vi "Send to HTTP Manager.vi"(8 "error in (no error)":errorcluster, 9 "Data":variant, 10 "ID":string, 11 "VolatusAPI in":refnum<class "VolatusAPI.lvclass">) -> (0 "error out":errorcluster, 3 "VolatusAPI out":refnum<class "VolatusAPI.lvclass">)   [LabVIEW 2020, in "Volatus.lvlib" / "VolatusAPI.lvclass"]
uses:
  VolatusAPI.lvclass
  VolatusAPI.lvclass/VolatusAPI.ctl
  MessageQ/MessageQ.lvclass
  HTTP Manager Identity/HTTP Manager Identity.lvclass
  C:/dev/lv20CE/relink/lv-volatus/Volatus/HTTP Manager Identity/HTTP Manager Identity.lvclass
  C:/dev/lv20CE/relink/lv-volatus/Volatus/Identity/Identity.lvclass
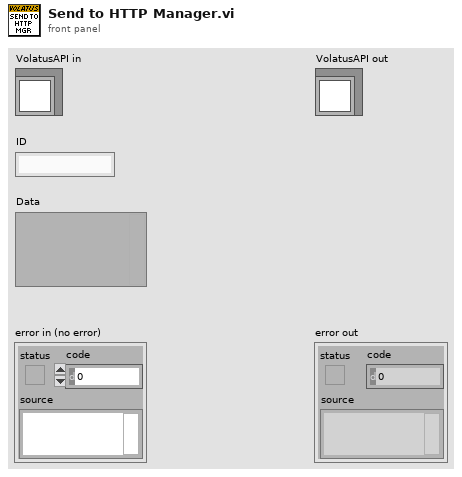
[diagram p1: front panel]
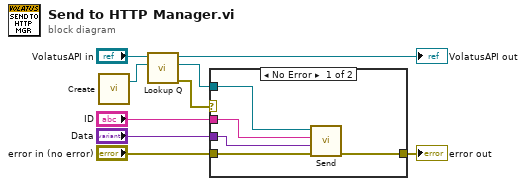
[diagram p0: block diagram]
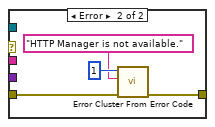
[diagram p2: hidden frame]
diagram:
  n1 = call "Create.vi"() -> ("HTTP Manager Identity out"=w9:refnum<class "HTTP Manager Identity.lvclass">)  [unwired: 7 in]
  n2 = call "Lookup Q.vi"("Identity"=w9, "VolatusAPI in"="VolatusAPI in") -> ("error out"=w8:errorcluster, "MessageQ"=w7:refnum<class "MessageQ.lvclass">, "VolatusAPI out"=→"VolatusAPI out":refnum<class "VolatusAPI.lvclass">)  [unwired: 7 in]
  n3 = case shown="No Error" w8 {
    tunnel: "error in (no error)" -> [w13 w18]
    tunnel: [w12 w17] -> w4
    tunnel: "Data" -> [w14 _]
    tunnel: w7 -> [w11 _]
    tunnel: "ID" -> [w10 _]
    frame No Error {
      n4 = call "Send.vi"("error in (no error)"=w13, "Data"=w14, "ID"=w10, "MessageQ in"=w11) -> ("error out"=w12:errorcluster)  [unwired: 6 in, 1 out]
    }
    frame Error {
      n5 = call <vilib>:"Error Cluster From Error Code.vi"("error in (no error)"=w18, "error message (\"\")"="HTTP Manager is not available.", "error code (0)"=1) -> ("error out"=w17:errorcluster)  [unwired: 6 in]
    }
  }
  "error out" <- w4
